vi "load_from_batch.vi"(0 "Base File Path":path=path "C:/data/RedMOT/2005.09.16", 1 "Base Filename":string="redMOTfreqj") -> (2 "atoms array":string[](array[string]), 3 "bkgnd array":string[](array[string]), 4 "Changed Values":dbl[](array[numeric]) format="%#_6f")   [LabVIEW 2013]
panel:
  out "path":path
  in  "dummy array":string[](array[string])
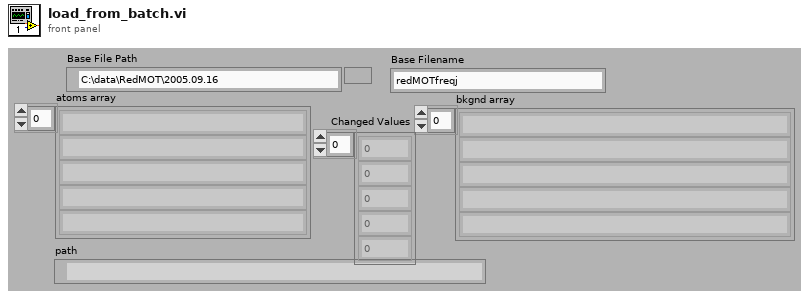
[diagram p1: front panel]
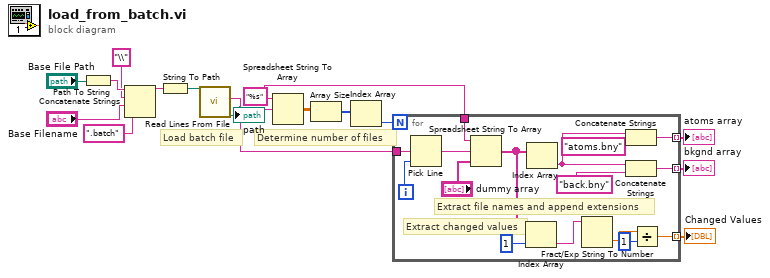
[diagram p0: block diagram]
diagram:
  w11 = "%s" ("format string")
  # "Determine number of files"
  # "Load batch file"
  n1 = Path To String(path="Base File Path") -> (string=w7:string)
  n2 = Concatenate Strings(w7, "\\", "Base Filename", ".batch" ("string")) -> (w5:string)
  n3 = String To Path(string=w5) -> (path=w6:path)
  "path" <- w6
  n4 = call <vilib>:"Read Lines From File.vi"("file path (dialog if empty)"=w6) -> ("line string"=w12:string)  [unwired: 5 in, 3 out]
  n5 = Spreadsheet String To Array(format string=w11, spreadsheet string=w12) -> (array=w15:dbl[][])  [unwired: 2 in]
  n6 = Array Size(array=w15) -> (size(s)=w14:i32[])
  n7 = Index Array(array=w14) -> (element=w13:i32)  [unwired: 1 in]
  n8 = for {
    N: w13 -> [_]
    tunnel: w12 -> [w31]
    tunnel: w11 -> [w28]
    tunnel: [w23] -> w10 mode=indexing
    tunnel: [w22] -> w9 mode=indexing
    tunnel: [w17] -> w1 mode=indexing
    i -> [w30]
    # "Extract changed values"
    # "Extract file names and append extensions"
    n9 = Pick Line(multi-line string=w31, line index=w30) -> (output string=w29:string)  [unwired: 1 in]
    n10 = Spreadsheet String To Array(format string=w28, spreadsheet string=w29, array type (2D Dbl)="dummy array") -> (array=w21:string[])  [unwired: 1 in]
    n11 = Index Array(array=w21, index=1) -> (element=w16:string)
    n12 = Index Array(array=w21) -> (element=w26:string)  [unwired: 1 in]
    n13 = Fract/Exp String To Number(string=w16) -> (number=w19:dbl)  [unwired: 3 in, 1 out]
    n14 = Concatenate Strings(w26, "atoms.bny" ("string")) -> (w22:string)
    n15 = Concatenate Strings(w26, "back.bny" ("string")) -> (w23:string)
    n16 = Divide(x=w19, y=1) -> (x/y=w17:dbl)
  }
  "bkgnd array" <- w10
  "atoms array" <- w9
  "Changed Values" <- w1
